vi "Rx Streaming Multi-Channel (Host).vi"() -> ()   [LabVIEW 2013]
doc: "This template is for the Simple NI-USRP Streaming design, a design that shows the basics of streaming data from an NI 294x/295x device. Refer to the block diagram for more information about how to use this template."
uses:
  <vilib>/userdefined/Silver/nirio_resource_slv.ctl
  SubVIs/Start Trigger.ctl
  <vilib>/Utility/error.llb/DialogType.ctl
  SubVIs/Configure Signal (Level).vi
panel:
  in  "reference level rf 1":dbl caption="Reference Level" format="%#_gdBm"
  in  "reference level rf 0":dbl caption="Reference Level" format="%#_gdBm"
  in  "lo frequency rf 1":dbl=-1.0 caption="LO Frequency" format="%#.3pHz"
  in  "lo frequency rf 0":dbl=-1.0 caption="LO Frequency" format="%#.3pHz"
  in  "frequency rf 1":dbl=2010000000.0 caption="Frequency" format="%#.3pHz"
  in  "frequency rf 0":dbl=1990000000.0 caption="Frequency" format="%#.3pHz"
  in  "antenna rf 1":string(combo)="RX1" caption="Active Antenna"
  in  "antenna rf 0":string(combo)="RX1" caption="Active Antenna"
  in  "enable rf 1":bool=TRUE
  in  "enable rf 0":bool=TRUE
  in  "reference frequency source":string(combo)="Internal" caption="Reference Frequency Source"
  in  "USRP RIO device":T1="RIO0" caption="USRP RIO Device"
  in  "number of samples is finite":bool=TRUE
  in  "sample rate":dbl=10000000.0 caption="Sample Rate" format="%#.3pS/s"
  in  "start trigger":T2=enum."Immediate" caption="Start Trigger"
  in  "tab control":T3(tab)
  out "Power Spectrum":cluster{"f0":dbl, "df":dbl, "magnitude":dbl[]}[](graph)
  out "Power Level":dbl[][](graph)
  out "I & Q Data":dbl[][](graph)
  in  "number of samples":u32=8192 caption="Number of Samples"
  in  "stop":bool
  # "Multi-Channel Rx Streaming"
  # "This template is for the Simple NI-USRP Streaming design, a design that shows the basics of streaming data from an NI 294x/295x device. See the block diagram for more information on how to use this template."
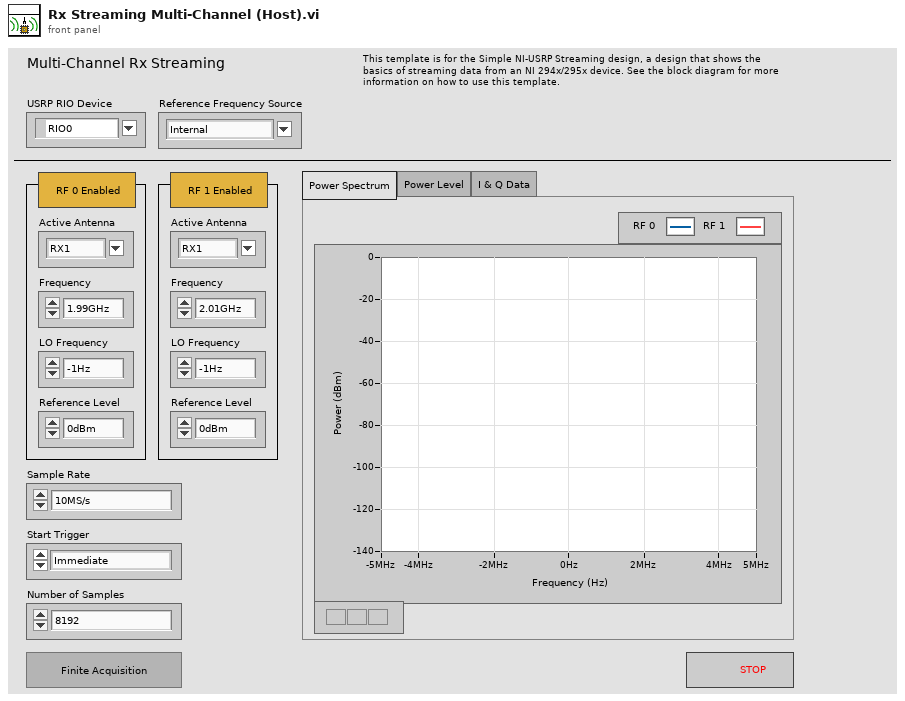
[diagram p1: front panel]
types:
  T1 = typedef "nirio_resource_slv.ctl" = tag
  T2 = typedef "Start Trigger.ctl" = enum8{"Software", "Digital Edge", "Rx Start Trigger", "Tx Start Trigger", "Immediate"}
  T3 = enum32{"Power Spectrum", "Power Level", "I & Q Data"}
  T4 = typedef "DialogType.ctl" = u16
  T5 = typedef "niUsrpRio Config v1 Host.lvlib/niUsrpRio Session.ctl" = cluster{"Global Settings Register Bus":T6, "Radio 0 Settings Register Bus":T6, "Rx NI-USRP session":refnum<k15>, "Tx NI-USRP session":refnum<k15>, "FPGA Interface":refnum<k20>, "RIO Interface Number":u32, "EEPROM Header":T7, "Device Data Header":T8, "EEPROM Characterization Header":T9, "Characterization Data":T10[], "Characterization Data Valid?":bool, "Radio 1 Settings Register Bus":T6, "Radio Settings Bus Semaphore":T12}
  T6 = typedef "niInstr Register Bus v0 Host.lvlib/Register Bus Session.ctl" = refnum<queue>
  T7 = typedef "niUsrpRio Config v1 Host.lvlib/EEPROM Header.ctl" = cluster{"Checksum":u32, "Product Code":u16, "Hardware Current Version":u16, "Hardware Oldest Compatible Version":u16, "EEPROM Map Current Version":u16, "EEPROM Map Oldest Compatible Version":u16, "User Password":string, "Pointer to Factory Header":u32, "Pointer to User Header":u32, "Recommended Interval":u16, "Number of Reserved Bytes":i32, "Number of Daughterboards":u8, "Daughterboard IDs":u16[], "Daughterboard Serial Numbers":string[]}
  T8 = typedef "niUsrpRio Config v1 Host.lvlib/EEPROM Device Data Header.ctl" = cluster{"Checksum":u32, "Number of Channels":u8, "Number of Gain Settings":u16[], "Pointer to Characterization Data":u32[], "Number of Reserved Bytes":i32, "Number of Frequencies":u16[]}
  T9 = typedef "niUsrpRio Config v1 Host.lvlib/EEPROM Characterization Header.ctl" = cluster{"Checksum":u32, "Date":timestamp, "Temperature":sgl, "Misc. Info":string, "Pointer to Device Data Header":u32, "Number of Reserved Bytes":i32}
  T10 = typedef "niUsrpRio Config v1 Host.lvlib/Characterization Data.ctl" = cluster{"Gains[dB]":dbl[], "Frequencies [Hz]":dbl[], "IQ Imbalance Table":T11[], "Measured Gains[dB]":dbl[][]}
  T11 = typedef "niUsrpRio Config v1 Host.lvlib/IQ Imbalance.ctl" = cluster{"Gain Imbalance [linear]":dbl, "Phase Imbalance [radians]":dbl, "Offset":cdb}
  T12 = typedef "Semaphore RefNum" = refnum<k1>
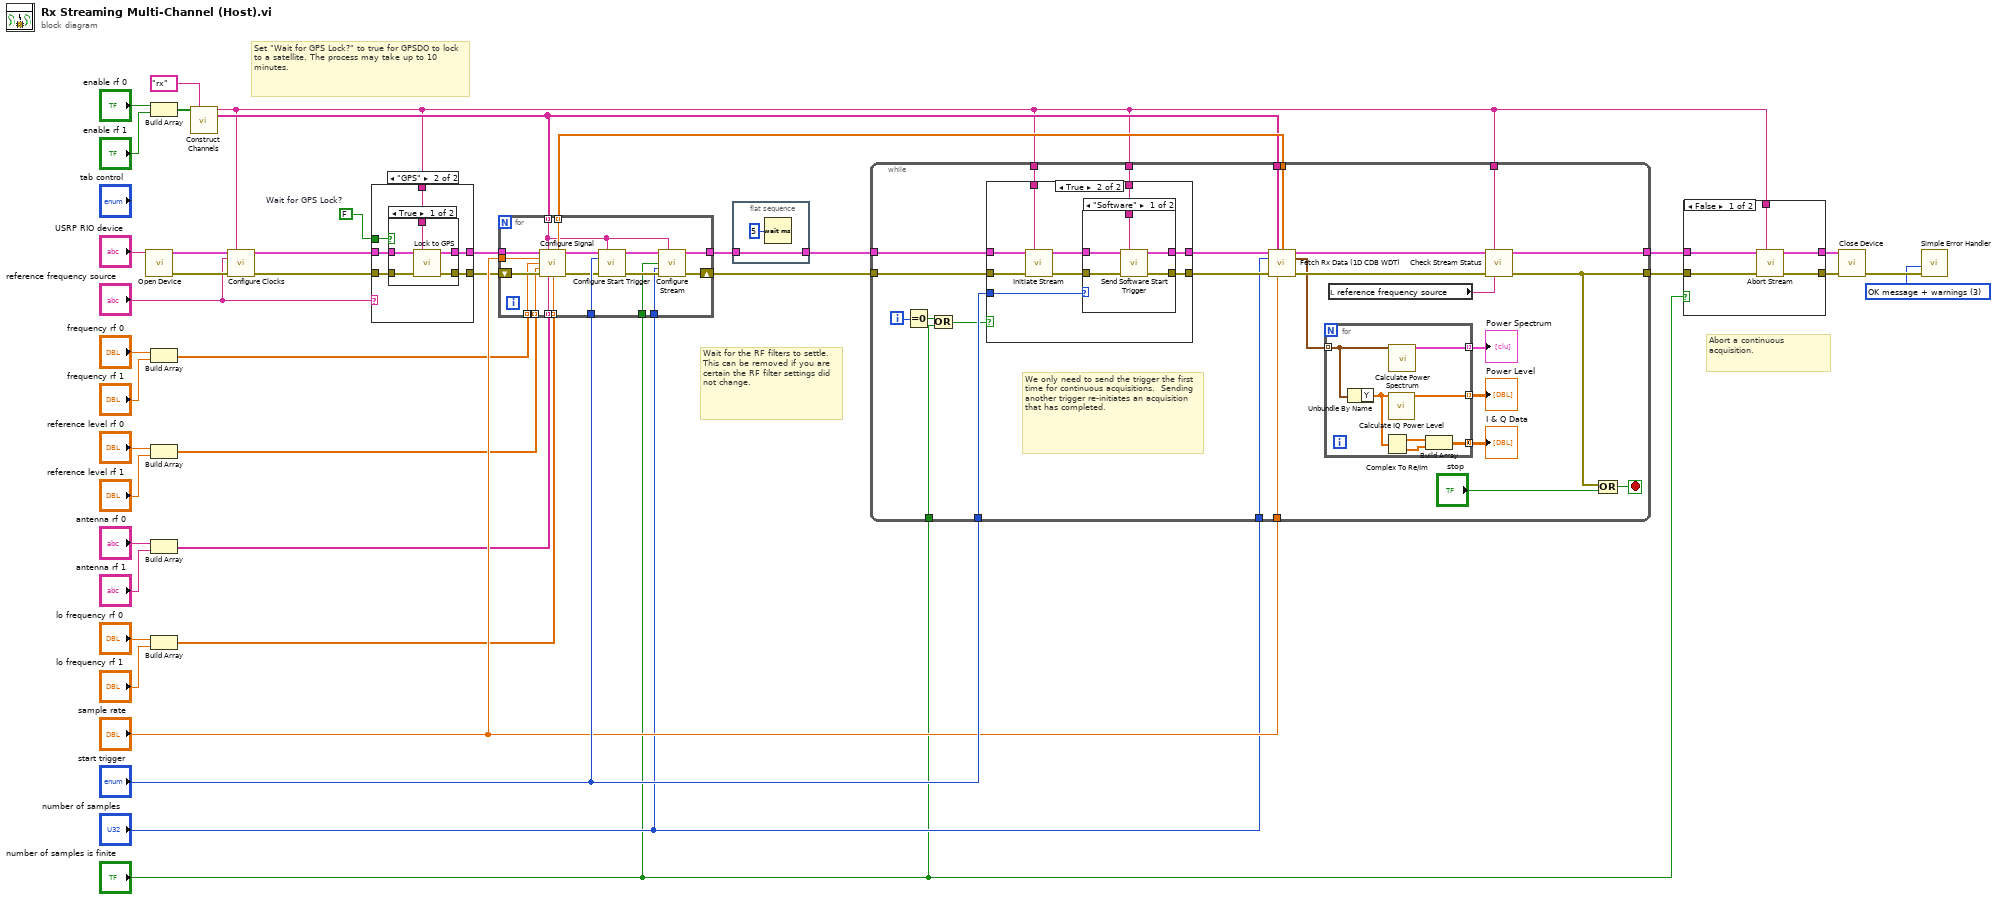
[diagram p0: block diagram]
diagram:
  w8 = FALSE  # Wait for GPS Lock?
  w39 = T4 3 items=["no dialog", "OK message", "continue or stop message", "OK message + warnings", "continue/stop + warnings"] ("type of dialog (OK msg:1)")
  # "Set \"Wait for GPS Lock?\" to true for GPSDO to lock to a satellite. The process may take up to 10 minutes."
  # "Wait for the RF filters to settle.  This can be removed if you are certain the RF filter settings did not change."
  # "Abort a continuous acquisition."
  n1 = call "Open Device.vi"("USRP RIO device"="USRP RIO device") -> ("niUsrpRio Session (out)"=w35:T5, "error out"=w34:errorcluster)  [unwired: 13 in]
  n2 = Build Array("enable rf 0", "enable rf 1") -> (w14:bool[])
  n3 = Build Array("frequency rf 0", "frequency rf 1") -> (w13:dbl[])
  n4 = Build Array("reference level rf 0", "reference level rf 1") -> (w12:dbl[])
  n5 = Build Array("antenna rf 0", "antenna rf 1") -> (w11:string[])
  n6 = Build Array("lo frequency rf 0", "lo frequency rf 1") -> (w10:dbl[])
  n7 = call "Construct Channels.vi"("enabled channels"=w14, "scope"="rx") -> ("scope"=w1:string, "channels"=w9:string[])  [unwired: 12 in]
  n8 = call "Configure Clocks.vi"("niUsrpRio Session"=w35, "scope"=w1, "Reference Frequency Source"="reference frequency source", "error in"=w34) -> ("niUsrpRio Session (out)"=w7:T5, "error out"=w6:errorcluster)  [unwired: 10 in]
  n9 = case shown="\"GPS\"" "reference frequency source" {
    tunnel: w7 -> [w43 w49]
    tunnel: [w43 w48] -> w5
    tunnel: [w42 w47] -> w4
    tunnel: w6 -> [w42 w46]
    tunnel: w1 -> [_ w45]
    tunnel: w8 -> [_ w44]
    frame Default {
    }
    frame "GPS" {
      n10 = case shown="True" w44 {
        tunnel: w49 -> [w51 w56]
        tunnel: [w54 w56] -> w48
        tunnel: [w53 w55] -> w47
        tunnel: w46 -> [w50 w55]
        tunnel: w45 -> [w52 _]
        frame True {
          n11 = call "Lock to GPS.vi"("niUsrpRio Session"=w51, "scope"=w52, "error in"=w50) -> ("niUsrpRio Session (out)"=w54:T5, "error out"=w53:errorcluster)  [unwired: 11 in]
        }
        frame False {
        }
      }
    }
  }
  n12 = for {
    tunnel: [w73] -> w38
    tunnel: "start trigger" -> [w72]
    tunnel: w5 -> [w66]
    tunnel: "sample rate" -> [w65]
    tunnel: [w64] -> w32 mode=indexing
    tunnel: "number of samples" -> [w63]
    tunnel: "number of samples is finite" -> [w62]
    shift-right: [w74] -> w41
    shift-left: w4 -> [w67]
    tunnel: w9 -> [w61] mode=indexing
    tunnel: w10 -> [w60] mode=indexing
    tunnel: w13 -> [w59] mode=indexing
    tunnel: w12 -> [w58] mode=indexing
    tunnel: w11 -> [w57] mode=indexing
    n13 = call-poly "Configure Signal.vi"("niUsrpRio Session"=w66, "scope"=w61, "sample rate [S/s]"=w65, "frequency [Hz]"=w59, "level [dBm]"=w58, "error in"=w67, "Active Antenna"=w57, "LO frequency [Hz]"=w60) -> ("coerced vertical range [Vpp]"=w64:dbl, "niUsrpRio Session (out)"=w69:T5, "error out"=w70:errorcluster)  [unwired: 1 in, 4 out]
    n14 = call "Configure Start Trigger.vi"("niUsrpRio Session"=w69, "scope"=w61, "start trigger"=w72, "error in"=w70) -> ("niUsrpRio Session (out)"=w68:T5, "error out"=w71:errorcluster)  [unwired: 10 in]
    n15 = call "Configure Stream.vi"("niUsrpRio Session"=w68, "scope"=w61, "number of samples is finite"=w62, "number of samples"=w63, "error in"=w71) -> ("niUsrpRio Session (out)"=w73:T5, "error out"=w74:errorcluster)  [unwired: 9 in]
  }
  n16 = flat-sequence {
    tunnel: w38 -> [w75]
    tunnel: [w75] -> w37
    frame #0 {
      # "Wait for the RF filters to settle.  This can be removed if you are certain the RF filter settings did not change."
      n17 = Wait (ms)(milliseconds to wait=u32 5) -> ()  [unwired: 1 out]
    }
  }
  n18 = while {
    tunnel: w37 -> [w94]
    tunnel: [w101] -> w30
    tunnel: w32 -> [w84]
    tunnel: "sample rate" -> [w90]
    tunnel: "number of samples" -> [w89]
    tunnel: "start trigger" -> [w97]
    tunnel: w41 -> [w96]
    tunnel: [w100] -> w29
    tunnel: "number of samples is finite" -> [w86]
    tunnel: w9 -> [w83]
    tunnel: w1 -> [w80]
    tunnel: w1 -> [w79]
    tunnel: w1 -> [w78]
    i -> [w87]
    stop <- w103 stop-if-true
    # "We only need to send the trigger the first time for continuous acquisitions.  Sending another trigger re-initiates an acquisition that has completed."
    # "Acquire and Fetch a waveform"
    n19 = Equal To 0?(x=w87) -> (x = 0?=w88:bool)
    n20 = Or(x=w88, y=w86) -> (x .or. y?=w85:bool)
    n21 = case shown="True" w85 {
      tunnel: w97 -> [_ w115]
      tunnel: w96 -> [w111 w117]
      tunnel: [w111 w121] -> w95
      tunnel: w94 -> [w112 w119]
      tunnel: [w112 w120] -> w93
      tunnel: w80 -> [_ w114]
      tunnel: w79 -> [_ w113]
      frame False {
      }
      frame True {
        n22 = call "Initiate Stream.vi"("niUsrpRio Session"=w119, "scope"=w114, "error in"=w117) -> ("niUsrpRio Session (out)"=w118:T5, "error out"=w116:errorcluster)  [unwired: 11 in]
        n23 = case shown="\"Software\"" w115 {
          tunnel: w116 -> [w126 w128]
          tunnel: w118 -> [w124 w127]
          tunnel: [w125 w128] -> w121
          tunnel: [w123 w127] -> w120
          tunnel: w113 -> [w122 _]
          frame "Software" {
            # "Send the software trigger to the master device only.  The master will also trigger all slave devices."
            n24 = call "Send Software Start Trigger.vi"("niUsrpRio Session"=w124, "scope"=w122, "error in"=w126) -> ("niUsrpRio Session (out)"=w123:T5, "error out"=w125:errorcluster)  [unwired: 11 in]
          }
          frame Default {
          }
        }
      }
    }
    n25 = call "Fetch Rx Data (1D CDB WDT).vi"("niUsrpRio Session"=w93, "scope"=w83, "vertical ranges [Vpp]"=w84, "number of samples"=w89, "error in"=w95, "sample rate"=w90) -> ("niUsrpRio Session (out)"=w91:T5, "Waveforms (CDB WDT)"=w82:waveform(cdb)[], "error out"=w92:errorcluster)  [unwired: 7 in]
    n26 = for {
      tunnel: [w110] -> w99 mode=indexing
      tunnel: [w109] -> w98 mode=concatenating
      tunnel: w82 -> [w104] mode=indexing
      tunnel: [w105] -> w81 mode=indexing
      n27 = Unbundle By Name(w104) -> ("Y"=w108:cdb[])
      n28 = Complex To Re/Im(x + iy=w108) -> (x=w107:dbl[], y=w106:dbl[])
      n29 = call "Calculate IQ Power Level.vi"("IQ data"=w108) -> ("power level (dBm)"=w110:dbl[])  [unwired: 14 in]
      n30 = call "Calculate Power Spectrum.vi"("IQ Waveform"=w104) -> ("power spectrum (dBm)"=w105:cluster{"f0":dbl, "df":dbl, "magnitude":dbl[]})  [unwired: 14 in]
      n31 = Build Array(w107, w106) -> (w109:dbl[][])
    }
    "Power Level" <- w99
    "Power Spectrum" <- w81
    "I & Q Data" <- w98
    n32 = local read "reference frequency source"() -> (w77:string)
    n33 = call "Check Stream Status.vi"("niUsrpRio Session"=w91, "scope"=w78, "error in"=w92, "reference frequency source"=w77) -> ("niUsrpRio Session (out)"=w101:T5, "error out"=w100:errorcluster)  [unwired: 9 in, 1 out]
    n34 = Or(x=w100, y="stop") -> (x .or. y?=w103:bool)
  }
  n35 = case shown="False" "number of samples is finite" {
    tunnel: w30 -> [w133 w135]
    tunnel: w29 -> [w132 w134]
    tunnel: [w131 w135] -> w28
    tunnel: [w130 w134] -> w27
    tunnel: w1 -> [w129 _]
    frame False {
      n36 = call "Abort Stream.vi"("niUsrpRio Session"=w133, "scope"=w129, "error in"=w132) -> ("niUsrpRio Session (out)"=w131:T5, "error out"=w130:errorcluster)  [unwired: 11 in]
    }
    frame True {
    }
  }
  n37 = call "Close Device.vi"("niUsrpRio Session"=w28, "error in"=w27) -> ("error out"=w40:errorcluster)  [unwired: 13 in]
  n38 = call <vilib>:"Simple Error Handler.vi"("type of dialog (OK msg:1)"=w39, "error in (no error)"=w40) -> ()  [unwired: 3 in, 5 out]
